vi "Read GoTo Reference.vi"(8 "error in (no error)":errorcluster, 11 "Skillbook in":refnum<class "Skillbook.lvclass">) -> (0 "error out":errorcluster, 2 "GoTo Reference":refnum<data-value>, 3 "Skillbook out":refnum<class "Skillbook.lvclass">)   [LabVIEW 2022 SP3, in "Skillbook.lvclass"]
uses:
  Skillbook.lvclass
  GoToSkill_class/GoToSkill.lvclass
  Skillbook.lvclass/Skillbook.ctl
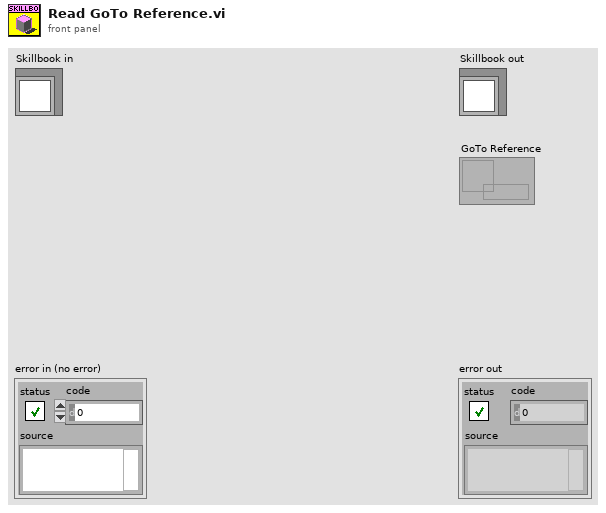
[diagram p1: front panel]
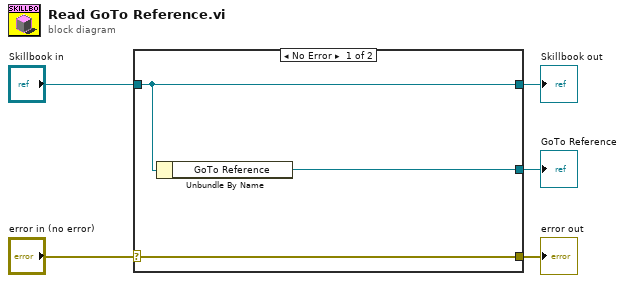
[diagram p0: block diagram]
diagram:
  n1 = case shown="No Error" "error in (no error)" {
    selector: "error in (no error)" -> [w8 w9]
    tunnel: [w8 w9] -> w4
    tunnel: [w7 w10] -> w2
    tunnel: "Skillbook in" -> [w7 w10]
    tunnel: [w6 _] -> w1
    frame No Error {
      n2 = Unbundle By Name(w7) -> ("GoTo Reference"=w6:refnum<data-value>)
    }
    frame Error {
    }
  }
  "error out" <- w4
  "Skillbook out" <- w2
  "GoTo Reference" <- w1
